vi "Auton Abort Global.vi"() -> ()   [LabVIEW 2016, in "Auton Mode Base.lvclass"]
uses:
  Auton Mode Base.lvclass
panel:
  in  "Abort Action":refnum<queue>
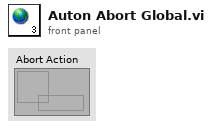
[diagram p1: front panel]
diagram:
